vi "Get Icon.vi"(8 "error in (no error)":errorcluster, 11 "Package in":refnum<class "Package.lvclass">) -> (0 "error out":errorcluster, 2 "Package Icon":picture, 3 "Package out":refnum<class "Package.lvclass">)   [LabVIEW 2020, in "GCentral-API.lvlib" / "Package.lvclass"]
uses:
  Package.lvclass
  Package.lvclass/Package.ctl
  GCentral-API.lvlib
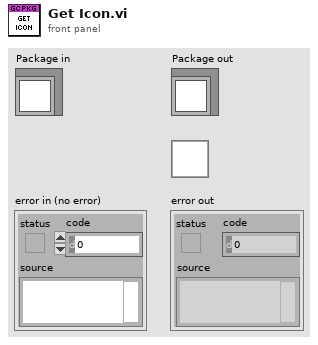
[diagram p1: front panel]
types:
  T1 = typedef "imagedata.ctl" = cluster{"image type":i32, "image depth":i32, "image":u8[], "mask":u8[], "colors":u32[], "Rectangle":cluster{"left":i16, "top":i16, "right":i16, "bottom":i16}}
  T2 = typedef "LVBoundsTypeDef.ctl" = cluster{"Width":u32, "Height":u32}
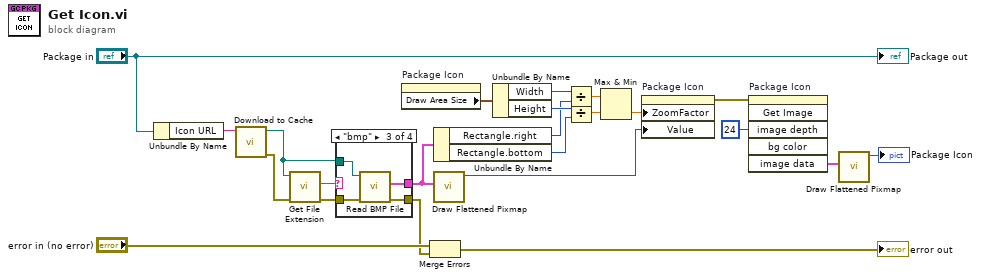
[diagram p0: block diagram]
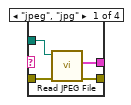
[diagram p2: hidden frame]
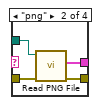
[diagram p3: hidden frame]
diagram:
  n1 = Unbundle By Name("Package in") -> ("Icon URL"=w20:string)
  n2 = call "Download to Cache.vi"("URL"=w20) -> ("error out"=w17:errorcluster, "Cache Path"=w16:path)  [unwired: 7 in, 2 out]
  n3 = call <vilib>:"Get File Extension.vi"("error in (no error)"=w17, "file"=w16) -> ("error out"=w18:errorcluster, "lowercase file extension"=w19:string)  [unwired: 5 in, 3 out]
  n4 = case shown="\"bmp\"" w19 {
    tunnel: w16 -> [w26 w31 w32 _]
    tunnel: w18 -> [w27 w30 w35 w36]
    tunnel: [w25 w29 w34 w36] -> w15
    tunnel: [w24 w28 w33 _] -> w13
    frame "jpeg", "jpg" {
      n5 = call <vilib>:"Read JPEG File.vi"("error in (no error)"=w27, "path to JPEG file"=w26) -> ("error out"=w25:errorcluster, "image data"=w24:T1)  [unwired: 7 in, 1 out]
    }
    frame "png" {
      n6 = call <vilib>:"Read PNG File.vi"("error in (no error)"=w30, "path to PNG file"=w31) -> ("error out"=w29:errorcluster, "image data"=w28:T1)  [unwired: 7 in, 1 out]
    }
    frame "bmp" {
      n7 = call <vilib>:"Read BMP File.vi"("error in (no error)"=w35, "path to BMP file"=w32) -> ("error out"=w34:errorcluster, "image data"=w33:T1)  [unwired: 7 in, 1 out]
    }
    frame Default {
    }
  }
  n8 = property on="Package Icon" class="Pict"() -> ("Draw Area Size"=w14:T2)  [unwired: 2 in, 2 out]
  n9 = Merge Errors("error in (no error)", w15) -> (→"error out":errorcluster)
  n10 = Unbundle By Name(w13) -> ("Rectangle.right"=w10:i16, "Rectangle.bottom"=w9:i16)
  n11 = call <vilib>:"Draw Flattened Pixmap.vi"("image data"=w13) -> ("new picture"=w3:picture)  [unwired: 1 in, 7 out]
  n12 = Unbundle By Name(w14) -> ("Width"=w12:u32, "Height"=w11:u32)
  n13 = Divide(x=w12, y=w10) -> (x/y=w8:dbl)
  n14 = Divide(x=w11, y=w9) -> (x/y=w7:dbl)
  n15 = Max & Min(x=w8, y=w7) -> (min(x,y)=w6:dbl)  [unwired: 1 out]
  n16 = property on="Package Icon" class="Pict"("ZoomFactor"=w6, "Value"=w3) -> (error out=w5:errorcluster)  [unwired: 2 in, 1 out]
  n17 = invoke on="Package Icon" class="Pict" method="Get Image"(error in=w5, "image depth"=24 ("Image Depth")) -> ("image data"=w4:T1)  [unwired: 4 in, 5 out]
  n18 = call <vilib>:"Draw Flattened Pixmap.vi"("image data"=w4) -> ("new picture"=→"Package Icon":picture)  [unwired: 1 in, 7 out]
  "Package out" <- "Package in"
